vi "LVClass_Camera read camera.vi"(8 "error in (no error)":errorcluster, 11 "Camera in":refnum<class "Camera.lvclass">) -> (0 "error out":errorcluster, 2 "ClassID_void":T1, 3 "Camera out":refnum<class "Camera.lvclass">)   [LabVIEW 2020, in "Camera.lvclass"]
uses:
  Camera.lvclass
  ClassID.ctl
  Camera.lvclass/Camera.ctl
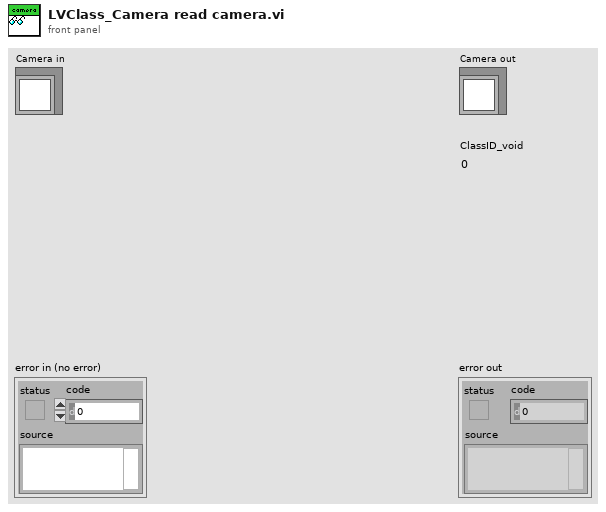
[diagram p1: front panel]
types:
  T1 = typedef "ClassID.ctl" = i64
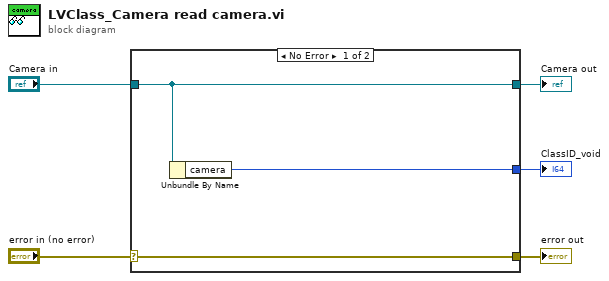
[diagram p0: block diagram]
diagram:
  n1 = case shown="No Error" "error in (no error)" {
    selector: "error in (no error)" -> [w8 w9]
    tunnel: [w8 w9] -> w4
    tunnel: [w7 w10] -> w2
    tunnel: "Camera in" -> [w7 w10]
    tunnel: [w6 _] -> w1
    frame No Error {
      n2 = Unbundle By Name(w7) -> ("camera"=w6:T1)
    }
    frame Error {
    }
  }
  "error out" <- w4
  "Camera out" <- w2
  "ClassID_void" <- w1
